vi "FA Graphic View.vi"() -> ()   [LabVIEW 2016, in "M1M3SupportEUI_Views.lvlib"]
uses:
  M1M3SupportEUI_Views.lvlib
  <vilib>/Math Plots/3D Math Plots/3D Scatter/3D Scatter XCtrl/3D Scatter.xctl
  Model/Model.lvclass
  SALLV_m1m3/DataTypes/ForceActuatorData.ctl
  <vilib>/Math Plots/3D Math Plots/3D Plot/3D Plot/Typedef/Sprite Type.ctl
  M1M3 Support Events/M1M3 Support Events.lvclass/M1M3 Support Events.ctl
  Typedefs/StateTypes.ctl
  <vilib>/Math Plots/3D Math Plots/3D Scatter/3D Scatter Datatype/Public/Plot Helper (Vector).vi
  <vilib>/Math Plots/3D Math Plots/3D Scatter/3D Scatter Datatype/3D Scatter Datatype.lvclass
  M1M3 Support Events/M1M3 Support Events.lvclass
  Typedefs/M1M3SupportEUI_TypeDefs.lvlib
  <vilib>/Math Plots/3D Math Plots/3D Plot/3D Plot/3D Plot.lvclass
  SALLV_m1m3/SALLV_m1m3.lvlib
panel:
  in  "ForceActuatorData":T1
  out "FA Data Time Stamp":timestamp
  in  "Data Type":string(combo)
  in  "Model in":refnum<class "Model.lvclass">
  out "3D Scatter":refnum<class "3D Plot Datatype.lvclass">[](xcontrol)
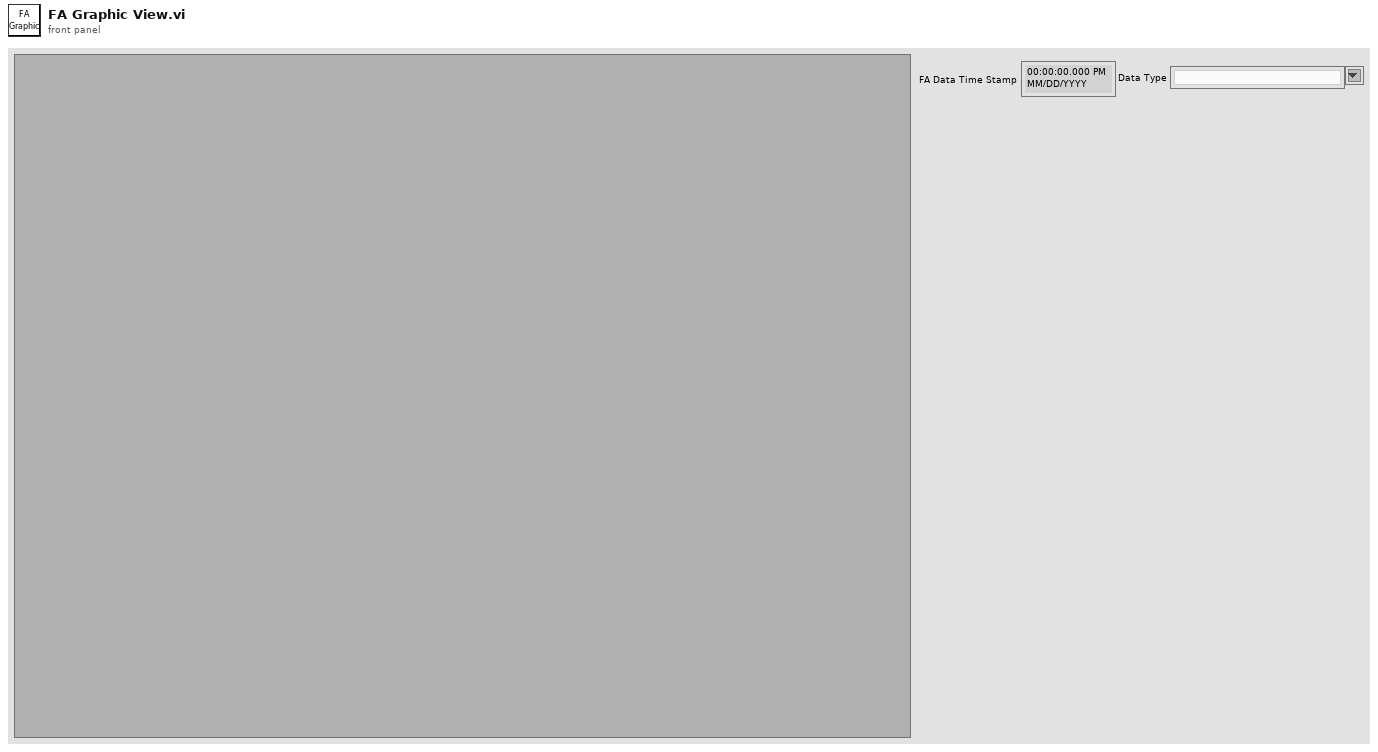
[diagram p1: front panel]
types:
  T1 = typedef "SALLV_m1m3.lvlib/ForceActuatorData.ctl" = cluster{"Timestamp":dbl, "StaticXSetpoint[156]":dbl[], "StaticYSetpoint[156]":dbl[], "StaticZSetpoint[156]":dbl[], "ElevationXSetpoint[156]":dbl[], "ElevationYSetpoint[156]":dbl[], "ElevationZSetpoint[156]":dbl[], "ElevationSetpointPercentage":dbl, "AzimuthXSetpoint[156]":dbl[], "AzimuthYSetpoint[156]":dbl[], "AzimuthZSetpoint[156]":dbl[], "TemperatureXSetpoint[156]":dbl[], "TemperatureYSetpoint[156]":dbl[], "TemperatureZSetpoint[156]":dbl[], "ActiveOpticsZSetpoint[156]":dbl[], "AberrationZSetpoint[156]":dbl[], "HardpointOffloadXSetpoint[156]":dbl[], "HardpointOffloadYSetpoint[156]":dbl[], "HardpointOffloadZSetpoint[156]":dbl[], "DynamicXSetpoint[156]":dbl[], "DynamicYSetpoint[156]":dbl[], "DynamicZSetpoint[156]":dbl[], "OffsetXSetpoint[156]":dbl[], "OffsetYSetpoint[156]":dbl[], "OffsetZSetpoint[156]":dbl[], "XSetpoint[156]":dbl[], "YSetpoint[156]":dbl[], "ZSetpoint[156]":dbl[], "PrimaryCylinderSetpointCommanded[156]":i32[], "SecondaryCylinderSetpointCommanded[156]":i32[], "BroadcastCounter[156]":u8[], "SlewFlagCommanded[156]":bool[], "PrimaryCylinderForce[156]":sgl[], "SecondaryCylinderForce[156]":sgl[], "ILCFault[156]":bool[], "DCAFault[156]":bool[], "XForce[156]":dbl[], "YForce[156]":dbl[], "ZForce[156]":dbl[]}
  T2 = typedef "3D Plot.lvclass/Sprite Type.ctl" = enum16{"None", "Empty Square", "Solid Square", "Empty Diamond", "Solid Diamond", "Empty Circle", "Solid Circle", "Asterisk", "Bold X", "Wireframe Sphere", "Solid Sphere", "Wireframe Cube", "Solid Cube"}
  T3 = typedef "M1M3SupportEUI_TypeDefs.lvlib/M1M3 Support Events.ctl" = cluster{"M1M3 Support State":refnum<user-event>, "Inclinometer  Data":refnum<user-event>, "IMS Data":refnum<user-event>, "FA Status":refnum<user-event>, "SAL Connected":refnum<user-event>, "HP Data":refnum<user-event>, "HP Status":refnum<user-event>, "Accelerometer Data":refnum<user-event>, "FPGA Data":refnum<user-event>, "Inclinometer Data":refnum<user-event>, "MirrorForces Data":refnum<user-event>, "OuterLoop Data":refnum<user-event>, "ErrorCode Event":refnum<user-event>, "InterlockStatus Event":refnum<user-event>, "InterlockWarning Event":refnum<user-event>, "FA Data":refnum<user-event>, "HPMonitorStatus Event":refnum<user-event>, "Gyro Data":refnum<user-event>}
  T4 = typedef "M1M3SupportEUI_TypeDefs.lvlib/StateTypes.ctl" = u32
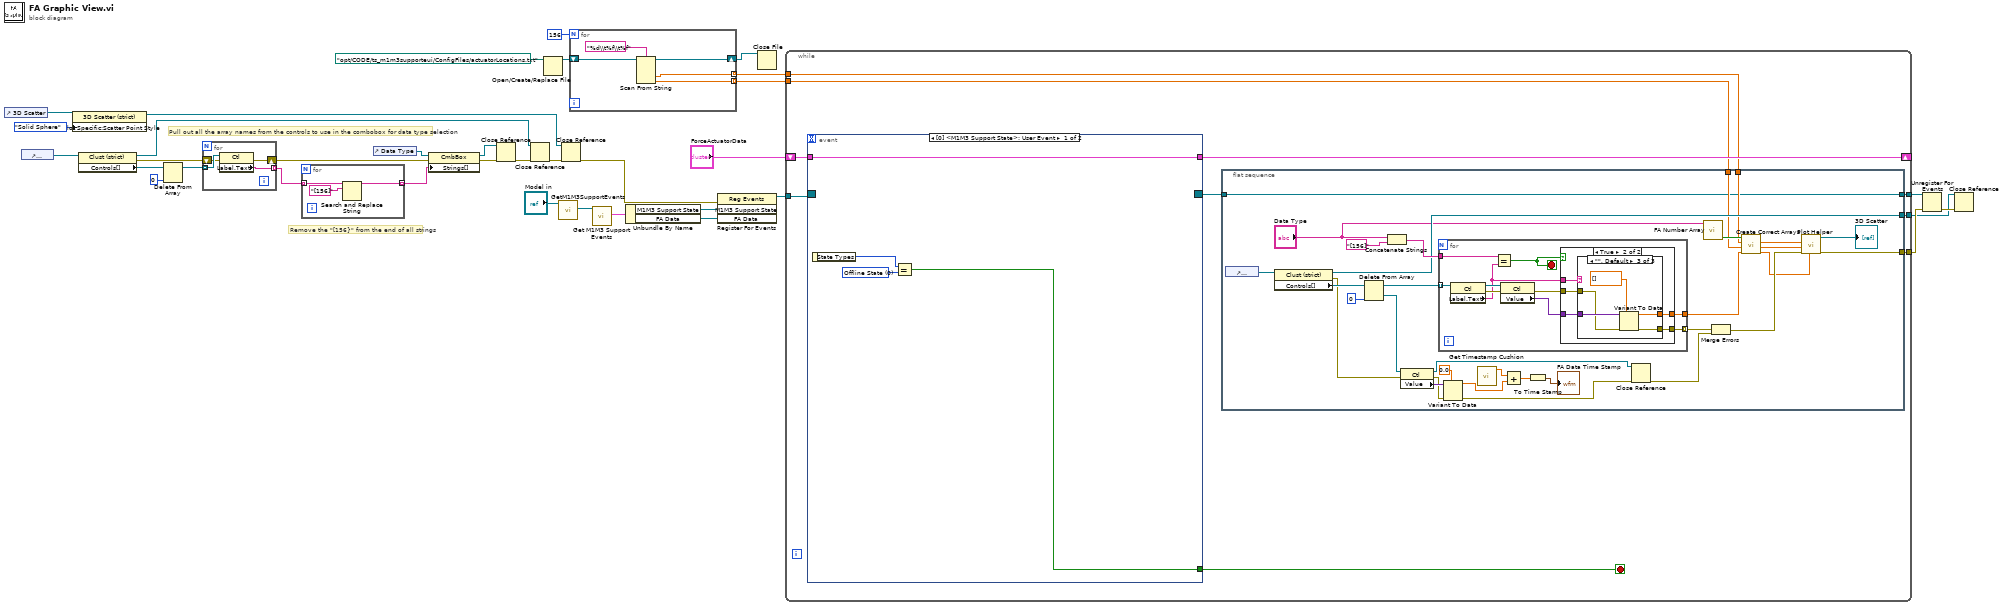
[diagram p0: block diagram]
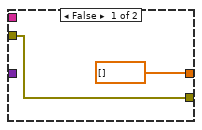
[diagram p2: hidden frame]
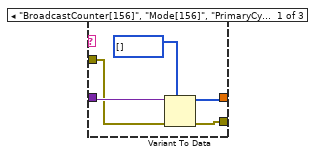
[diagram p3: hidden frame]
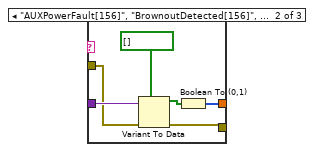
[diagram p4: hidden frame]
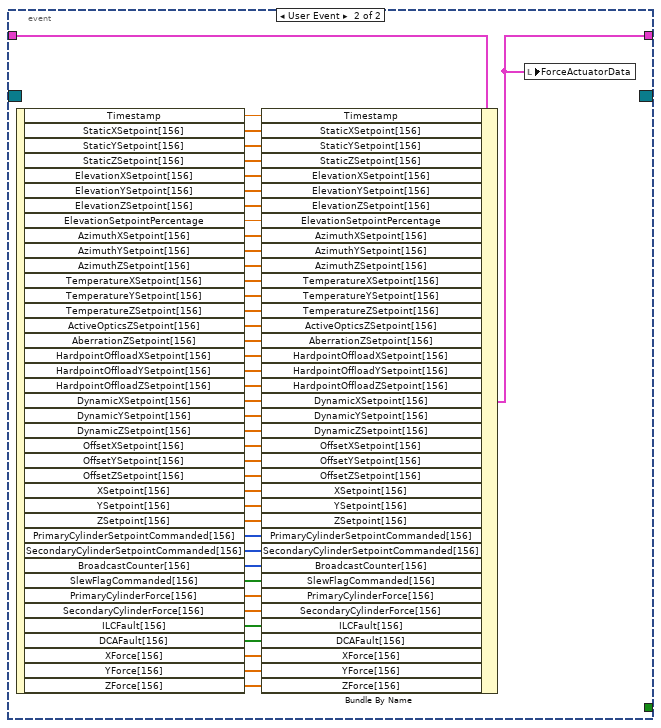
[diagram p5: hidden frame]
diagram:
  # "Remove the \"[156}\" from the end of all strings"
  # "Pull out all the array names from the controls to use in the combobox for data type selection"
  n1 = control-ref of="3D Scatter"() -> (w4:refnum<vi>)
  n2 = control-ref of="ForceActuatorData"() -> (w16:refnum<vi>)
  n3 = property class="3D Scatter (strict)"(reference=w4, "Plot Specific:Scatter Point Style"=Sprite_Type."Solid Sphere" ("Plot Specific:Scatter:Scatter Point Style")) -> (reference out=w1:refnum<vi>)  [unwired: 1 in, 1 out]
  n4 = property class="Clust (strict)"(reference=w16) -> (reference out=w12:refnum<vi>, error out=w17:errorcluster, "Controls[]"=w20:refnum<vi>[])  [unwired: 1 in]
  n5 = Delete From Array(array=w20, index=0) -> (array with subset deleted=w21:refnum<vi>[])  [unwired: 1 in, 1 out]
  n6 = for {
    tunnel: w21 -> [w39] mode=indexing
    tunnel: [w38] -> w18 mode=indexing
    shift-right: [w36] -> w23
    shift-left: w17 -> [w37]
    n7 = property class="Ctl"(reference=w39, error in=w37) -> (error out=w36:errorcluster, "Label.Text"=w38:string)  [unwired: 1 out]
  }
  n8 = for {
    tunnel: w18 -> [w42] mode=indexing
    tunnel: [w41] -> w19 mode=indexing
    n9 = Search and Replace String(input string=w42, search string="[156]") -> (result string=w41:string)  [unwired: 6 in, 3 out]
  }
  n10 = control-ref of="Data Type"() -> (w11:refnum<vi>)
  n11 = property class="CmbBox"(reference=w11, error in=w23, "Strings[]"=w19) -> (reference out=w14:refnum<vi>, error out=w15:errorcluster)
  n12 = Close Reference(reference=w14, error in (no error)=w15) -> (error out=w13:errorcluster)
  n13 = Close Reference(reference=w12, error in (no error)=w13) -> (error out=w3:errorcluster)
  n14 = Open/Create/Replace File(file path (use dialog)=path "/opt/CODE/ts_m1m3supporteui/ConfigFiles/actuatorLocations.txt") -> (refnum out=w34:refnum<file>)  [unwired: 5 in, 2 out]
  n15 = call "GetM1M3SupportEvents.vi"("Model in"="Model in") -> ("M1M3 Support Events out"=w31:refnum<class "M1M3 Support Events.lvclass">)  [unwired: 8 in, 2 out]
  n16 = Close Reference(reference=w1, error in (no error)=w3) -> (error out=w2:errorcluster)
  n17 = for {
    N: 156 -> [_]
    shift-right: [w45] -> w33
    shift-left: w34 -> [w47]
    tunnel: [w44] -> w10 mode=indexing
    tunnel: [w43] -> w9 mode=indexing
    n18 = Scan From String("%d\\t%f\\t%f" ("format string"), w47) -> (w45:refnum<file>, output 2=w44:dbl, output 3=w43:dbl)  [unwired: 5 in, 1 out]
  }
  n19 = call "Get M1M3 Support Events.vi"("M1M3 Support Events in"=w31) -> ("M1M3 Support Events"=w29:T3)  [unwired: 9 in, 1 out]
  n20 = Unbundle By Name(w29) -> ("M1M3 Support State"=w30:refnum<user-event>, "FA Data"=w25:refnum<user-event>)
  n21 = register-events(error in=w2, w30, w25) -> (reference out=w27:refnum<event-registration>)  [unwired: 1 in, 1 out]
  n22 = Close File(refnum=w33) -> ()  [unwired: 1 in, 2 out]
  n23 = while {
    tunnel: w27 -> [w57]
    tunnel: [w48] -> w26
    shift-right: [w54] -> _
    shift-left: "ForceActuatorData" -> [w55]
    tunnel: w10 -> [w51]
    tunnel: w9 -> [w50]
    tunnel: [w53] -> w8
    tunnel: [w52] -> w6
    stop <- w56 stop-if-true
    n24 = event shown="[0] <M1M3 Support State>: User Event" {
      selector: w57 -> [_ _]
      dyn-events: [_ _] -> w49
      timeout: _ -> [_ _]
      tunnel: [w124 _] -> w56
      tunnel: w55 -> [w123 w167]
      tunnel: [w123 w127] -> w54
      event User Event {
        w126 = T4 0 items=["Offline State"=0, "Fault State"=4294967295, "Standby State"=16777216, "Disabled State"=33554432, "Enabled State"=50331648, "Parked State"=50331649, "Raising State"=50331650, "Active State"=50331651, "Lowering State"=50331652, "Engineering State"=50397184, "Parked Engineering State"=50397185, "Raising Engineering State"=50397186, "Active Engineering State"=50397187, "Lowering Engineering State"=50397188] ("y")
        n25 = event-data() -> ("State Types"=w125:T4)  [unwired: 1 in]
        n26 = Equal?(x=w125, y=w126) -> (x = y?=w124:bool)
      }
      event User Event {
        n27 = event-data() -> ("Timestamp"=w166:dbl, "StaticXSetpoint[156]"=w165:dbl[], "StaticYSetpoint[156]"=w164:dbl[], "StaticZSetpoint[156]"=w163:dbl[], "ElevationXSetpoint[156]"=w162:dbl[], "ElevationYSetpoint[156]"=w161:dbl[], "ElevationZSetpoint[156]"=w160:dbl[], "ElevationSetpointPercentage"=w159:dbl, "AzimuthXSetpoint[156]"=w158:dbl[], "AzimuthYSetpoint[156]"=w157:dbl[], "AzimuthZSetpoint[156]"=w156:dbl[], "TemperatureXSetpoint[156]"=w155:dbl[], "TemperatureYSetpoint[156]"=w154:dbl[], "TemperatureZSetpoint[156]"=w153:dbl[], "ActiveOpticsZSetpoint[156]"=w152:dbl[], "AberrationZSetpoint[156]"=w151:dbl[], "HardpointOffloadXSetpoint[156]"=w150:dbl[], "HardpointOffloadYSetpoint[156]"=w149:dbl[], "HardpointOffloadZSetpoint[156]"=w148:dbl[], "DynamicXSetpoint[156]"=w147:dbl[], "DynamicYSetpoint[156]"=w146:dbl[], "DynamicZSetpoint[156]"=w145:dbl[], "OffsetXSetpoint[156]"=w144:dbl[], "OffsetYSetpoint[156]"=w143:dbl[], "OffsetZSetpoint[156]"=w142:dbl[], "XSetpoint[156]"=w141:dbl[], "YSetpoint[156]"=w140:dbl[], "ZSetpoint[156]"=w139:dbl[], "PrimaryCylinderSetpointCommanded[156]"=w138:i32[], "SecondaryCylinderSetpointCommanded[156]"=w137:i32[], "BroadcastCounter[156]"=w136:u8[], "SlewFlagCommanded[156]"=w135:bool[], "PrimaryCylinderForce[156]"=w134:sgl[], "SecondaryCylinderForce[156]"=w133:sgl[], "ILCFault[156]"=w132:bool[], "DCAFault[156]"=w131:bool[], "XForce[156]"=w130:dbl[], "YForce[156]"=w129:dbl[], "ZForce[156]"=w128:dbl[])  [unwired: 1 in]
        n28 = Bundle By Name(cluster=w167, "Timestamp"=w166, "StaticXSetpoint[156]"=w165, "StaticYSetpoint[156]"=w164, "StaticZSetpoint[156]"=w163, "ElevationXSetpoint[156]"=w162, "ElevationYSetpoint[156]"=w161, "ElevationZSetpoint[156]"=w160, "ElevationSetpointPercentage"=w159, "AzimuthXSetpoint[156]"=w158, "AzimuthYSetpoint[156]"=w157, "AzimuthZSetpoint[156]"=w156, "TemperatureXSetpoint[156]"=w155, "TemperatureYSetpoint[156]"=w154, "TemperatureZSetpoint[156]"=w153, "ActiveOpticsZSetpoint[156]"=w152, "AberrationZSetpoint[156]"=w151, "HardpointOffloadXSetpoint[156]"=w150, "HardpointOffloadYSetpoint[156]"=w149, "HardpointOffloadZSetpoint[156]"=w148, "DynamicXSetpoint[156]"=w147, "DynamicYSetpoint[156]"=w146, "DynamicZSetpoint[156]"=w145, "OffsetXSetpoint[156]"=w144, "OffsetYSetpoint[156]"=w143, "OffsetZSetpoint[156]"=w142, "XSetpoint[156]"=w141, "YSetpoint[156]"=w140, "ZSetpoint[156]"=w139, "PrimaryCylinderSetpointCommanded[156]"=w138, "SecondaryCylinderSetpointCommanded[156]"=w137, "BroadcastCounter[156]"=w136, "SlewFlagCommanded[156]"=w135, "PrimaryCylinderForce[156]"=w134, "SecondaryCylinderForce[156]"=w133, "ILCFault[156]"=w132, "DCAFault[156]"=w131, "XForce[156]"=w130, "YForce[156]"=w129, "ZForce[156]"=w128) -> (w127:T1)
        n29 = local write "ForceActuatorData"(w127) -> ()
      }
    }
    n30 = flat-sequence {
      tunnel: [w72] -> w53
      tunnel: [w71] -> w52
      tunnel: w51 -> [w68]
      tunnel: w50 -> [w66]
      tunnel: w49 -> [w62]
      tunnel: [w62] -> w48
      frame #0 {
        n31 = control-ref of="ForceActuatorData"() -> (w84:refnum<vi>)
        n32 = property class="Clust (strict)"(reference=w84) -> (reference out=w71:refnum<vi>, error out=w78:errorcluster, "Controls[]"=w83:refnum<vi>[])  [unwired: 1 in]
        n33 = Delete From Array(array=w83, index=0) -> (deleted portion=w79:refnum<vi>, array with subset deleted=w87:refnum<vi>[])  [unwired: 1 in]
        n34 = Concatenate Strings("Data Type", "[156]" ("string")) -> (w85:string)
        n35 = property class="Ctl"(reference=w79, error in=w78) -> (reference out=w82:refnum<vi>, error out=w77:errorcluster, "Value"=w81:variant)
        n36 = for {
          tunnel: [w98] -> w64
          tunnel: w85 -> [w91]
          tunnel: w87 -> [w97] mode=indexing
          tunnel: [w92] -> w75 mode=indexing
          stop <- w94 stop-if-true
          n37 = property class="Ctl"(reference=w97) -> (reference out=w95:refnum<vi>, error out=w96:errorcluster, "Label.Text"=w90:string)  [unwired: 1 in]
          n38 = Equal?(x=w91, y=w90) -> (x = y?=w94:bool)
          n39 = property class="Ctl"(reference=w95, error in=w96) -> (error out=w93:errorcluster, "Value"=w99:variant)  [unwired: 1 out]
          n40 = case shown="True" w94 {
            tunnel: w99 -> [_ w106]
            tunnel: [dbl[] [] w105] -> w98
            tunnel: w90 -> [_ w104]
            tunnel: w93 -> [w100 w103]
            tunnel: [w100 w102] -> w92
            frame False {
            }
            frame True {
              n41 = case shown="\"\", Default" w104 {
                tunnel: w106 -> [w110 w116 w122]
                tunnel: [w109 w114 w120] -> w105
                tunnel: w103 -> [w108 w113 w119]
                tunnel: [w107 w112 w118] -> w102
                frame "BroadcastCounter[156]", "Mode[156]", "PrimaryCylinderSetpointCommanded[156]", "SecondaryCylinderSetpointCommanded[156]" {
                  n42 = Variant To Data(error in=w108, type=i32[] [], Variant=w110) -> (data=w109:i32[], error out=w107:errorcluster)
                }
                frame "AUXPowerFault[156]", "BrownoutDetected[156]", "DCAAmplifierAFault[156]", "DCAAmplifierBFault[156]", "DCAEventTrapReset[156]", "DCAFault[156]", "DCAOutputsEnabled[156]", "DCAPowerFault[156]", "EventTrapReset[156]", "FaultOverridden[156]", "ILCFault[156]", "MajorFault[156]", "MinorFault[156]", "MotorPowerFault[156]", "SMCPowerFault[156]", "SSRPowerFault[156]", "SlewFlagCommanded[156]", "WatchdogReset[156]" {
                  n43 = Variant To Data(error in=w113, type=bool[] [], Variant=w116) -> (data=w115:bool[], error out=w112:errorcluster)
                  n44 = Boolean To (0,1)(Boolean=w115) -> (0, 1=w114:i16[])
                }
                frame "", Default {
                  n45 = Variant To Data(error in=w119, type=dbl[] [], Variant=w122) -> (data=w120:dbl[], error out=w118:errorcluster)
                }
              }
            }
          }
        }
        n46 = Variant To Data(error in=w77, type=0.0, Variant=w81) -> (data=w59:dbl, error out=w76:errorcluster)
        n47 = call "Get Timestamp Cushion.vi"() -> ("TimestampCushion"=w61:dbl)  [unwired: 11 in]
        n48 = Add(x=w61, y=w59) -> (x+y=w60:dbl)
        n49 = To Time Stamp(1:w60) -> (0:→"FA Data Time Stamp":timestamp)
        n50 = Close Reference(reference=w82, error in (no error)=w76) -> (error out=w74:errorcluster)
        n51 = call "FA Number Array.vi"("Data Type"="Data Type") -> ("On/Off Array"=w69:bool[])  [unwired: 9 in, 1 out]
        n52 = Merge Errors(w75, w74) -> (w73:errorcluster)
        n53 = call "Create Correct Arrays.vi"("Data"=w64, "YCoordinates"=w66, "XCoordinates"=w68, "UseActuatorArray"=w69) -> ("NewData"=w63:dbl[], "NewYCoordinates"=w65:dbl[], "NewXCoordinates"=w67:dbl[])  [unwired: 5 in]
        n54 = call-poly <vilib>:"Plot Helper.vi"("z vector"=w63, "error in (no error)"=w73, "y vector"=w65, "x vector"=w67) -> ("error out"=w72:errorcluster, "3D Plot lvclass Array out"=→"3D Scatter":refnum<class "3D Plot Datatype.lvclass">[])  [unwired: 2 in, 4 out]
      }
    }
  }
  n55 = Unregister For Events(event registration refnum=w26, error in=w8) -> (error out=w7:errorcluster)
  n56 = Close Reference(reference=w6, error in (no error)=w7) -> ()  [unwired: 1 out]
